vi "Assert ExcuseNote.vi"() -> ()   [LabVIEW 2015, in "Member_Actor.lvlib" / "ExcuseNote.lvclass"]
uses:
  ExcuseNote.lvclass
  API/_Database/Database.lvclass
  ExcuseNote.lvclass/ExcuseNote.ctl
  Member_Actor.lvlib
panel:
  in  "CurWeek(0)":i32=7
  in  "Name(\"\")":string="钱凌峰"
  in  "ID(\"\")":string="1110810220"
  in  "path":path=path "E:/哈工大竞技机器人队/机器人队管理系统/Database/CRTDatabase.accdb"
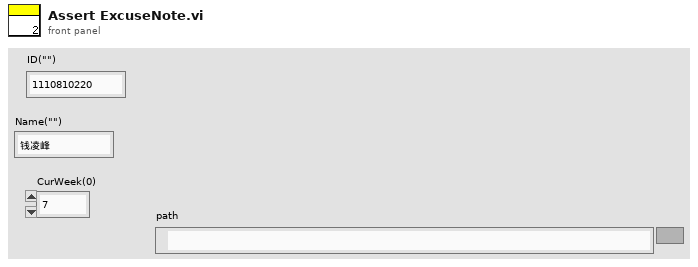
[diagram p1: front panel]
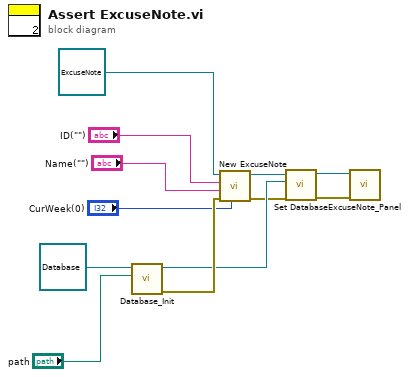
[diagram p0: block diagram]
diagram:
  n1 = call "Database_Init.vi"("path"="path", "object in"=refnum<class "Database.lvclass"> refnum ("Database")) -> ("error out"=w4:errorcluster, "object out"=w3:refnum<class "Database.lvclass">)  [unwired: 8 in]
  n2 = call "New ExcuseNote.vi"("CurWeek(0)"="CurWeek(0)", "error in (no error)"=w4, "Name(\"\")"="Name(\"\")", "ID(\"\")"="ID(\"\")", "ExcuseNote in"=refnum<class "ExcuseNote.lvclass"> refnum ("Member_Actor.lvlib:ExcuseNote.lvclass")) -> ("error out"=w2:errorcluster, "ExcuseNote out"=w7:refnum<class "ExcuseNote.lvclass">)  [unwired: 5 in]
  n3 = call "Set Database.vi"("error in (no error)"=w2, "Database"=w3, "ExcuseNote in"=w7) -> ("error out"=w11:errorcluster, "ExcuseNote out"=w12:refnum<class "ExcuseNote.lvclass">)  [unwired: 7 in]
  n4 = call "ExcuseNote_Panel.vi"("error in (no error)"=w11, "PanelController"=w12) -> ()  [unwired: 8 in, 2 out]
